vi "Module Identities.vi"(8 "error in (no error)":errorcluster, 11 "Remote Messaging Module in":refnum<class "Remote Messaging Module.lvclass">) -> (0 "error out":errorcluster, 2 "Identities":refnum<class "Identity.lvclass">[](array[class]), 3 "Remote Messaging Module out":refnum<class "Remote Messaging Module.lvclass">)   [LabVIEW 2020, in "Volatus.lvlib" / "Remote Messaging Module.lvclass"]
uses:
  Remote Messaging Module.lvclass
  Identity/Identity.lvclass
  Remote Messaging Identity/Remote Messaging Identity.lvclass
  C:/dev/lv20CE/relink/lv-volatus/Volatus/Identity/Identity.lvclass
  Remote Messaging Module.lvclass/Remote Messaging Module.ctl
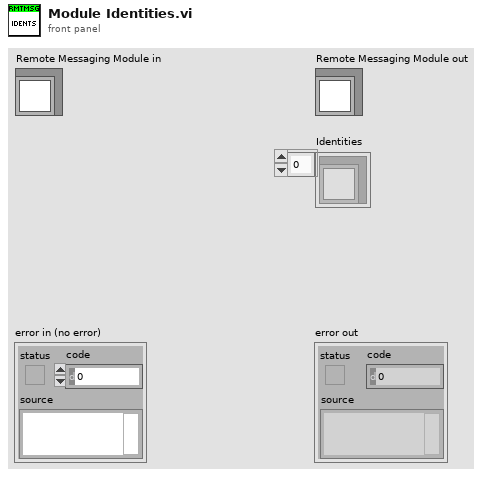
[diagram p1: front panel]
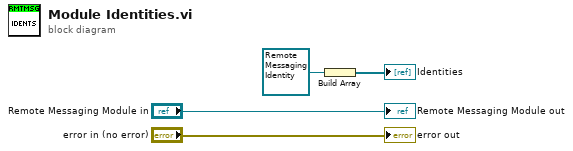
[diagram p0: block diagram]
diagram:
  n1 = Build Array(refnum<class "Remote Messaging Identity.lvclass"> refnum ("Volatus:Remote Messaging Identity.lvclass")) -> (→"Identities":refnum<class "Remote Messaging Identity.lvclass">[])
  "error out" <- "error in (no error)"
  "Remote Messaging Module out" <- "Remote Messaging Module in"
